vi "GetActualShoulderAngleData.vi"(11 "Reset Encoder":bool) -> (2 "Encoder Speed (deg/s)":dbl, 3 "Encoder Angle (deg)":dbl)   [LabVIEW 2018]
uses:
  <vilib>/Rock Robotics/Network Tables/NT Write Number.vi
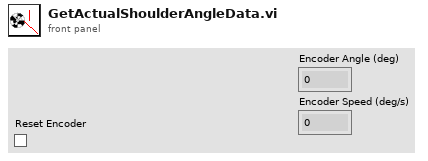
[diagram p1: front panel]
types:
  T1 = typedef "WPI_EncoderDevRef.ctl" = cluster{"DevStatus":errorcluster, "EncoderIndex":T2, "CounterIndex":T3, "DistancePerCount":dbl, "Decoding Type":T4}
  T2 = typedef "FPGA_EncoderIdx.ctl" = enum8{"Enc 0", "Enc 1", "Enc 2", "Enc 3", "Enc 4", "Enc 5", "Enc 6", "Enc 7", "Invalid"}
  T3 = typedef "FPGA_CounterCtrSystemIndex.ctl" = enum8{"Ctr 0", "Ctr 1", "Ctr 2", "Ctr 3", "Ctr 4", "Ctr 5", "Ctr 6", "Ctr 7", "Invalid"}
  T4 = typedef "WPI_EncoderType.ctl" = enum16{"1x", "2x", "4x"}
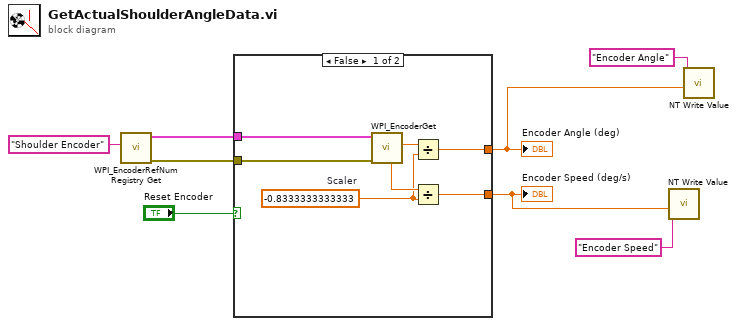
[diagram p0: block diagram]
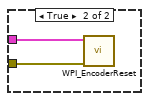
[diagram p2: hidden frame]
diagram:
  n1 = call <vilib>:"WPI_EncoderRefNum Registry Get.vi"("refnum name"="Shoulder Encoder") -> ("error out"=w6:errorcluster, "EncoderDevRef"=w8:T1)  [unwired: 9 in]
  n2 = case shown="False" "Reset Encoder" {
    tunnel: w8 -> [w15 w17]
    tunnel: w6 -> [w14 w16]
    tunnel: [w10 _] -> w2
    tunnel: [w9 _] -> w4
    frame False {
      w11 = -0.8333333333333  # Scaler
      n3 = call <vilib>:"WPI_EncoderGet.vi"("error in (no error)"=w14, "EncoderDevRef"=w15) -> ("Distance"=w13:dbl, "Rate"=w12:dbl)  [unwired: 4 in, 4 out]
      n4 = Divide(x=w13, y=w11) -> (x/y=w10:dbl)
      n5 = Divide(x=w12, y=w11) -> (x/y=w9:dbl)
    }
    frame True {
      n6 = call <vilib>:"WPI_EncoderReset.vi"("error in (no error)"=w16, "EncoderDevRef"=w17) -> ()  [unwired: 8 in, 2 out]
    }
  }
  "Encoder Angle (deg)" <- w2
  "Encoder Speed (deg/s)" <- w4
  n7 = call-poly <vilib>:"NT Write Value.vi"("Numeric"=w4, "Name"="Encoder Speed") -> ()  [unwired: 9 in, 1 out]
  n8 = call-poly <vilib>:"NT Write Value.vi"("Numeric"=w2, "Name"="Encoder Angle") -> ()  [unwired: 9 in, 1 out]
